vi "Turret_Execute.vi"() -> ()   [LabVIEW 2019]
uses:
  Globals/Turret_Globals.vi
  <vilib>/Rock Robotics/WPI/ThirdParty/Phoenix-LabVIEW/Motor Controller/Controls/CTRE_Phoenix_MotorControl_ControlMode.ctl
panel:
  out "Turret_Control_Mode":T1 items=["PercentOutput"=0, "Position"=1, "Velocity"=2, "Current"=3, "Follower"=5, "MotionProfile"=6, "MotionMagic"=7, "MotionProfileArc"=10, "Disabled"=15]
  out "Turret_Spin_Speed":dbl
  out "Flywheel_Control_Mode":T1 items=["PercentOutput"=0, "Position"=1, "Velocity"=2, "Current"=3, "Follower"=5, "MotionProfile"=6, "MotionMagic"=7, "MotionProfileArc"=10, "Disabled"=15]
  out "Flywheel_Speed":dbl
  in  "turret_spin_encoder":dbl
  in  "t_x":dbl
  in  "Kp Aim":dbl=0.08
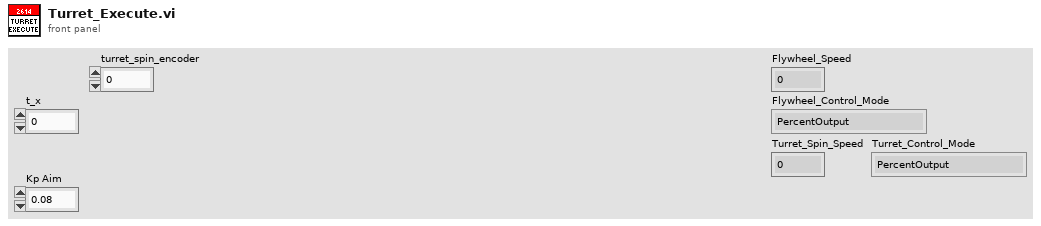
[diagram p1: front panel]
types:
  T1 = typedef "CTRE_Phoenix_MotorControl_ControlMode.ctl" = u16
  T2 = typedef "Turret_Cluster.ctl" = cluster{"Auto-Target?":bool, "Control_State":enum16{"Manual_Percent_Voltage", "Manual_Speed_Control", "Auto-Target"}, "Turret_Spin_Speed":dbl, "Flywheel_Speed":dbl, "Flywheel_Speed_Control?":bool, "Turret_Spin_Speed_Control?":bool}
  T3 = enum16{"Manual_Percent_Voltage", "Manual_Speed_Control", "Auto-Target"}
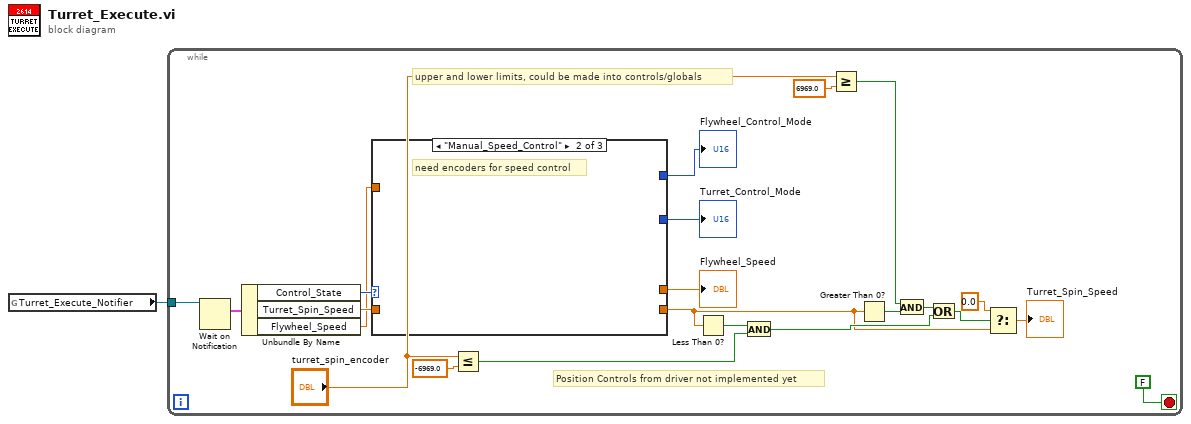
[diagram p0: block diagram]
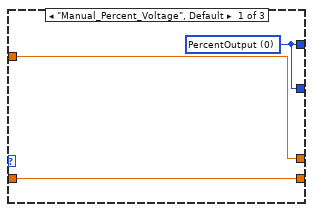
[diagram p2: hidden frame]
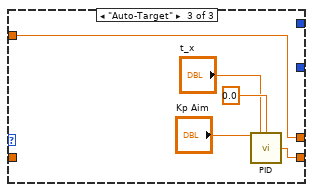
[diagram p3: hidden frame]
diagram:
  n1 = global read "Turret_Globals.vi" "Turret_Execute_Notifier"() -> (w1:refnum<notifier>)
  n2 = while {
    tunnel: w1 -> [w22]
    stop <- FALSE stop-if-true
    # "Position Controls from driver not implemented yet"
    # "upper and lower limits, could be made into controls/globals"
    n3 = Wait on Notification(notifier=w22) -> (notification=w21:T2)  [unwired: 3 in, 3 out]
    n4 = Unbundle By Name(w21) -> ("Control_State"=w20:T3, "Turret_Spin_Speed"=w19:dbl, "Flywheel_Speed"=w18:dbl)
    n5 = case shown="\"Manual_Speed_Control\"" w20 {
      tunnel: w19 -> [w26 _ _]
      tunnel: w18 -> [w25 _ w30]
      tunnel: [w26 _ w29] -> w6
      tunnel: [w25 _ w30] -> w17
      tunnel: [w24 _ _] -> w16
      tunnel: [w24 _ _] -> w15
      frame "Manual_Percent_Voltage", Default {
        w24 = T1 0 items=["PercentOutput"=0, "Position"=1, "Velocity"=2, "Current"=3, "Follower"=5, "MotionProfile"=6, "MotionMagic"=7, "MotionProfileArc"=10, "Disabled"=15] ("Control Mode")
      }
      frame "Manual_Speed_Control" {
        # "need encoders for speed control"
      }
      frame "Auto-Target" {
        n6 = call "PID.vi"("Kp"="Kp Aim", "Process Variable"="t_x", "Goal"=0.0) -> ("Command"=w29:dbl)  [unwired: 10 in, 2 out]
      }
    }
    "Flywheel_Speed" <- w17
    "Flywheel_Control_Mode" <- w15
    "Turret_Control_Mode" <- w16
    n7 = Less Or Equal?(x="turret_spin_encoder", y=-6969.0) -> (x <= y?=w12:bool)
    n8 = Less Than 0?(x=w6) -> (x < 0?=w11:bool)
    n9 = And(x=w11, y=w12) -> (x .and. y?=w10:bool)
    n10 = Greater Or Equal?(x="turret_spin_encoder", y=6969.0) -> (x >= y?=w14:bool)
    n11 = Greater Than 0?(x=w6) -> (x > 0?=w13:bool)
    n12 = And(x=w14, y=w13) -> (x .and. y?=w9:bool)
    n13 = Or(x=w9, y=w10) -> (x .or. y?=w8:bool)
    n14 = Select(t=0.0, s=w8, f=w6) -> (s? t:f=→"Turret_Spin_Speed":dbl)
  }
